vi "Run_Pre Core.vi"(0 "functionbase in":refnum<class "functionbase.lvclass">, 11 "error in (no error)":errorcluster) -> (4 "functionbase out":refnum<class "functionbase.lvclass">, 6 "Execute Run Core?":bool, 15 "error out":errorcluster)   [LabVIEW 2019, in "LSL.lvlib" / "functionbase.lvclass"]
uses:
  functionbase.lvclass
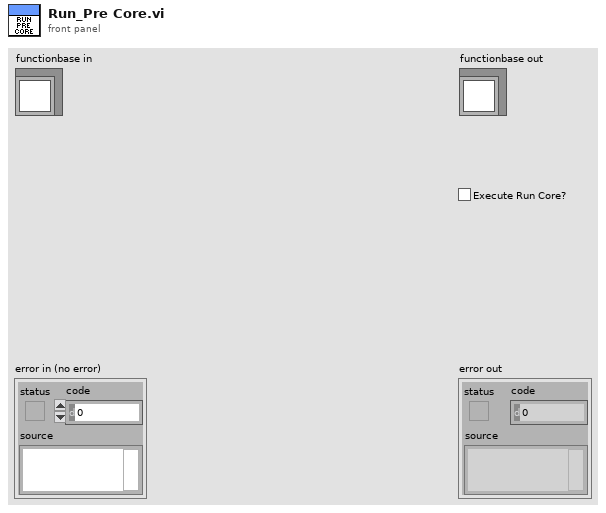
[diagram p1: front panel]
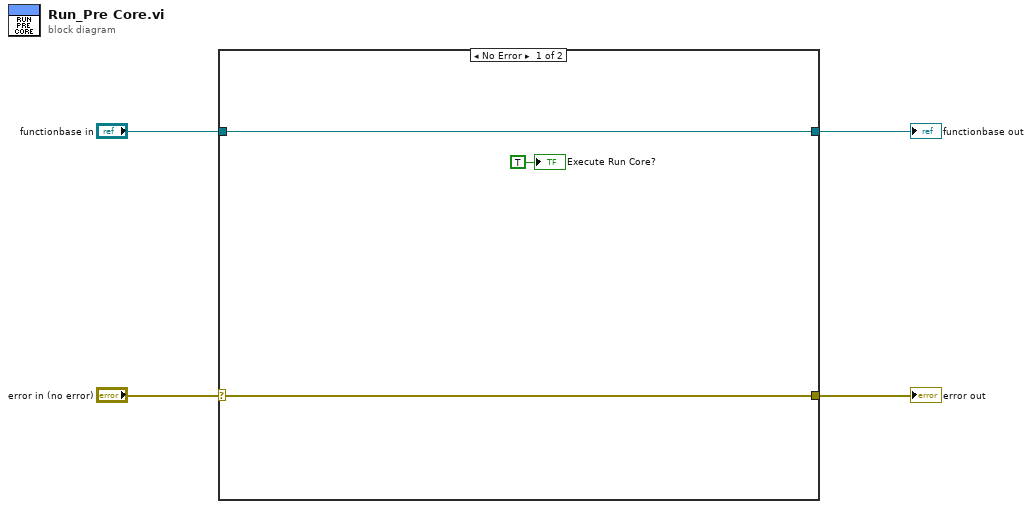
[diagram p0: block diagram]
diagram:
  n1 = case shown="No Error" "error in (no error)" {
    selector: "error in (no error)" -> [w6 w9]
    tunnel: [w6 w9] -> w3
    tunnel: [w7 w8] -> w1
    tunnel: "functionbase in" -> [w7 w8]
    frame No Error {
      "Execute Run Core?" <- TRUE ("Execute Run Core?")
    }
    frame Error {
    }
  }
  "error out" <- w3
  "functionbase out" <- w1
